vi "getCompleted.vi"(8 "error in (no error)":errorcluster, 11 "SudukuState in":refnum<class "SudukuState.lvclass">) -> (0 "error out":errorcluster, 2 "completed":i32, 3 "SudukuState out":refnum<class "SudukuState.lvclass">)   [LabVIEW 2009]
uses:
  SudukuState.lvclass
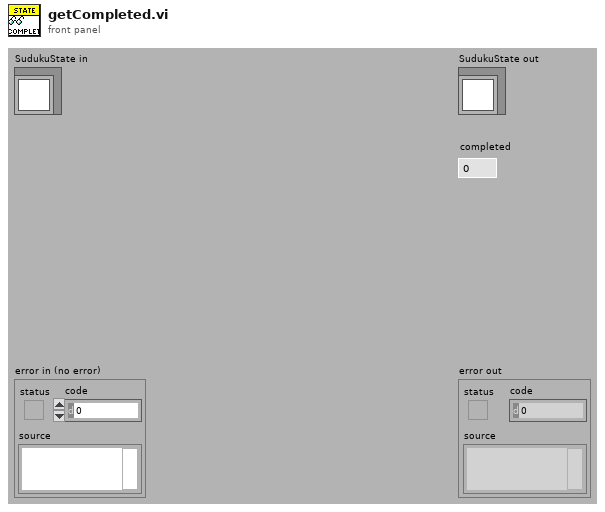
[diagram p1: front panel]
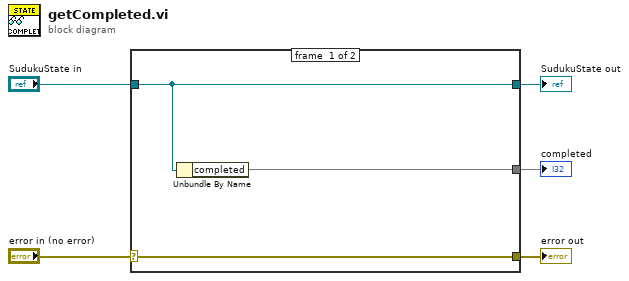
[diagram p0: block diagram]
diagram:
  n1 = case shown="No Error" "error in (no error)" {
    selector: "error in (no error)" -> [w8 w9]
    tunnel: [w8 w9] -> w4
    tunnel: [w7 w10] -> w2
    tunnel: "SudukuState in" -> [w7 w10]
    tunnel: [w6 _] -> w1
    frame #0 {
      n2 = Unbundle By Name(w7) -> ("completed"=w6)
    }
    frame #1 {
    }
  }
  "error out" <- w4
  "SudukuState out" <- w2
  "completed" <- w1
